vi "CheckFaults.vi"(11 "Axis":refnum<k21>) -> (0 "error out":errorcluster, 1 "Numeric":dbl)   [LabVIEW 2017, in "SoftmotionAxis.lvclass"]
uses:
  SoftmotionAxis.lvclass
  <resource>/objmgr/nimcai.rc
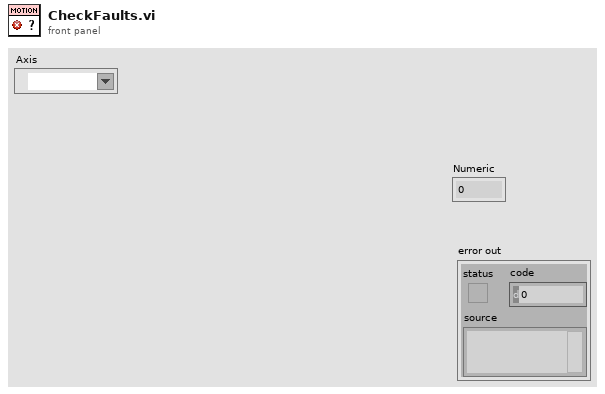
[diagram p1: front panel]
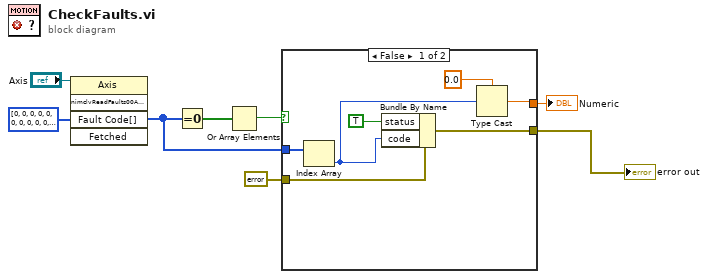
[diagram p0: block diagram]
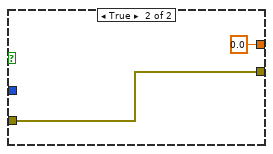
[diagram p2: hidden frame]
diagram:
  n1 = invoke class="Axis" method="nimclvReadFaults00A10001"(reference="Axis", "Fault Code[]"=i32[] [0, 0, 0, 0, 0, 0, 0, 0, 0, 0, 0]) -> ("Fault Code[]"=w2:i32[])  [unwired: 3 in, 4 out]
  n2 = Equal To 0?(x=w2) -> (x = 0?=w5:bool[])
  n3 = Or Array Elements(Boolean array=w5) -> (logical OR=w4:bool)
  n4 = case shown="False" w4 {
    tunnel: errorcluster {"status"=FALSE, "code"=0, "source"=""} ("error in (no error) 2") -> [w15 w17]
    tunnel: w2 -> [w14 _]
    tunnel: [w12 w17] -> w8
    tunnel: [w11 0.0] -> w1
    frame False {
      n5 = Index Array(array=w14) -> (element=w10:i32)  [unwired: 1 in]
      n6 = Bundle By Name(cluster=w15, "status"=TRUE, "code"=w10) -> (w12:errorcluster)
      n7 = Type Cast(type=0.0 ("Numeric"), x=w10) -> (*(type *) &x=w11:dbl)
    }
    frame True {
    }
  }
  "error out" <- w8
  "Numeric" <- w1
